vi "Test Configuration - SParam.vi"(8 "error in":errorcluster, 10 "Test Configuration":T2={"Action"=enum."Measure", "Pulse Mode"={"Pulse Mode Enabled"=FALSE, "Pulse Period (s)"=0.0, "Pulse Modulator Delay (s)"=0.0, "Pulse Modulator Width (s)"=0.0, "Pulse Acquisition Auto"=FALSE, "Pulse Acquisition Delay (s)"=0.0, "Pulse Acquisition Width (s)"=0.0}, "Frequency Sweep"={"Start Frequency (Hz)"=0.0, "Stop Frequency (Hz)"=0.0, "Number of Points"=0}, "S-Parameters"=[], "Magnitude Units"=0, "Phase Trace Type"=0, "SnP File Path"="", "Averaging Enabled"=FALSE, "Averaging Count"=10} {"Phase Trace Type" items=["Wrapped", "Unwrapped"]; "Pulse Mode"."Pulse Acquisition Width (s)" format="%.2p"; "Pulse Mode"."Pulse Acquisition Delay (s)" format="%.2p"; "Pulse Mode"."Pulse Modulator Width (s)" format="%.2p"; "Pulse Mode"."Pulse Modulator Delay (s)" format="%.2p"; "Pulse Mode"."Pulse Period (s)" format="%.2p"; "Magnitude Units" items=["dB", "Linear"]; "Frequency Sweep"."Stop Frequency (Hz)" format="%.3p"; "Frequency Sweep"."Start Frequency (Hz)" format="%.3p"}, 11 "RFmxVNA Session in":refnum<k21>) -> (0 "error out":errorcluster, 2 "S-Parameters":T1(array[cluster]), 3 "RFmxVNA Session out":refnum<k21>)   [LabVIEW 2023]
uses:
  Controls/Test Config - SParam.ctl
  <resource>/objmgr/RFmxVNA.rc
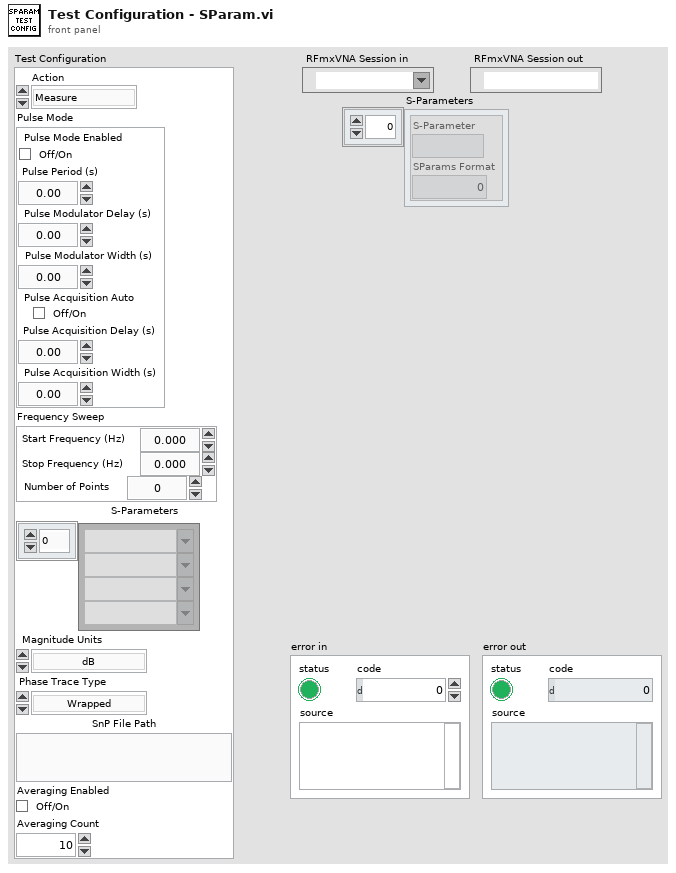
[diagram p1: front panel]
types:
  T1 = cluster{"S-Parameter":string, "SParams Format":i32}[]
  T2 = typedef "Test Config - SParam.ctl" = cluster{"Action":enum16{"Calibrate", "Measure"}, "Pulse Mode":cluster{"Pulse Mode Enabled":bool, "Pulse Period (s)":dbl, "Pulse Modulator Delay (s)":dbl, "Pulse Modulator Width (s)":dbl, "Pulse Acquisition Auto":bool, "Pulse Acquisition Delay (s)":dbl, "Pulse Acquisition Width (s)":dbl}, "Frequency Sweep":cluster{"Start Frequency (Hz)":dbl, "Stop Frequency (Hz)":dbl, "Number of Points":i32}, "S-Parameters":string[], "Magnitude Units":i32, "Phase Trace Type":i32, "SnP File Path":string, "Averaging Enabled":bool, "Averaging Count":u32}
  T3 = cluster{"S-Parameter":string, "SParams Format":i32}
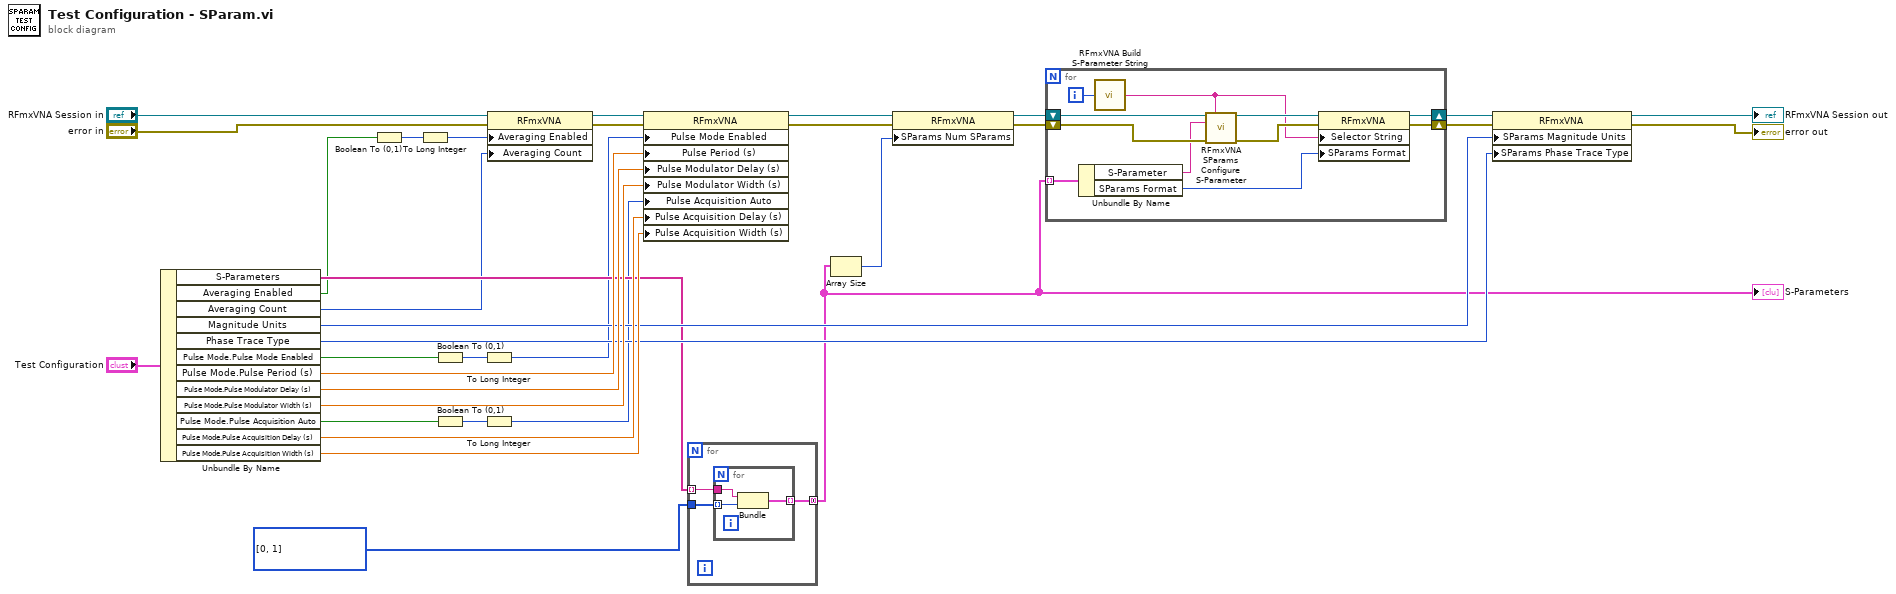
[diagram p0: block diagram]
diagram:
  w15 = i32[] [0, 1] items=["Magnitude", "Phase", "Complex", "SWR", "Smith Impedance", "Smith Admittance", "Polar"]
  n1 = Unbundle By Name("Test Configuration") -> ("S-Parameters"=w14:string[], "Averaging Enabled"=w8:bool, "Averaging Count"=w6:u32, "Magnitude Units"=w22:i32, "Phase Trace Type"=w23:i32, "Pulse Mode.Pulse Mode Enabled"=w26:bool, "Pulse Mode.Pulse Period (s)"=w27:dbl, "Pulse Mode.Pulse Modulator Delay (s)"=w28:dbl, "Pulse Mode.Pulse Modulator Width (s)"=w29:dbl, "Pulse Mode.Pulse Acquisition Auto"=w30:bool, "Pulse Mode.Pulse Acquisition Delay (s)"=w31:dbl, "Pulse Mode.Pulse Acquisition Width (s)"=w32:dbl)
  n2 = Boolean To (0,1)(Boolean=w8) -> (0, 1=w7:i16)
  n3 = To Long Integer(number=w7) -> (32bit integer=w5:i32)
  n4 = Boolean To (0,1)(Boolean=w26) -> (0, 1=w4:i16)
  n5 = Boolean To (0,1)(Boolean=w30) -> (0, 1=w3:i16)
  n6 = To Long Integer(number=w4) -> (32bit integer=w2:i32)
  n7 = To Long Integer(number=w3) -> (32bit integer=w1:i32)
  n8 = property class="RFmxVNA"(reference="RFmxVNA Session in", error in="error in", "Averaging Enabled"=w5, "Averaging Count"=w6) -> (reference out=w11:refnum<k21>, error out=w10:errorcluster)
  n9 = property class="RFmxVNA"(reference=w11, error in=w10, "Pulse Mode Enabled"=w2, "Pulse Period (s)"=w27, "Pulse Modulator Delay (s)"=w28, "Pulse Modulator Width (s)"=w29, "Pulse Acquisition Auto"=w1, "Pulse Acquisition Delay (s)"=w31, "Pulse Acquisition Width (s)"=w32) -> (reference out=w24:refnum<k21>, error out=w25:errorcluster)
  n10 = for {
    tunnel: w14 -> [w36] mode=indexing
    tunnel: w15 -> [w37]
    tunnel: [w35] -> w13 mode=concatenating
    n11 = for {
      tunnel: w37 -> [w39] mode=indexing
      tunnel: w36 -> [w40]
      tunnel: [w38] -> w35 mode=indexing
      n12 = Bundle("S-Parameter"=w40, "SParams Format"=w39) -> (w38:T3)  [unwired: 1 in]
    }
  }
  "S-Parameters" <- w13
  n13 = Array Size(array=w13) -> (size(s)=w18:i32)
  n14 = property class="RFmxVNA"(reference=w24, error in=w25, "SParams Num SParams"=w18) -> (reference out=w16:refnum<k21>, error out=w17:errorcluster)
  n15 = for {
    shift-right: [w51] -> w20
    shift-left: w17 -> [w49]
    shift-right: [w50] -> w19
    shift-left: w16 -> [w46]
    tunnel: w13 -> [w43] mode=indexing
    i -> [w48]
    n16 = Unbundle By Name(w43) -> ("S-Parameter"=w42:string, "SParams Format"=w41:i32)
    n17 = call <vilib>:"RFmxVNA Build S-Parameter String.vi"("S-Parameter Number"=w48) -> ("Selector String Out"=w44:string)  [unwired: 14 in]
    n18 = call <vilib>:"RFmxVNA SParams Configure S-Parameter.vi"("Instrument Handle In"=w46, "Selector String"=w44, "S-Parameter"=w42, "error in (no error)"=w49) -> ("Instrument Handle Out"=w45:refnum<k21>, "error out"=w47:errorcluster)  [unwired: 10 in]
    n19 = property class="RFmxVNA"(reference=w45, error in=w47, "Selector String"=w44, "SParams Format"=w41) -> (reference out=w50:refnum<k21>, error out=w51:errorcluster)
  }
  n20 = property class="RFmxVNA"(reference=w19, error in=w20, "SParams Magnitude Units"=w22, "SParams Phase Trace Type"=w23) -> (reference out=→"RFmxVNA Session out":refnum<k21>, error out=→"error out":errorcluster)
